vi "Server_Refresh Training Data.vi"(8 "error in":errorcluster, 11 "Index":i32) -> (0 "error out":errorcluster, 3 "Training Data":T1[](array[typedef]))   [LabVIEW 2018, in "Cloud Server.lvlib"]
uses:
  Cloud Server.lvlib
  Data Def/Server_Training Data.ctl
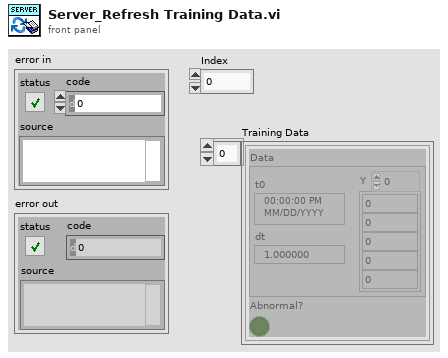
[diagram p1: front panel]
types:
  T1 = typedef "Cloud Server.lvlib/Server_Training Data.ctl" = cluster{"Data":waveform(dbl), "Abnormal?":bool}
  T2 = typedef "Cloud Server.lvlib/Server_Connection Properties.ctl" = cluster{"User Data":T3, "Data":waveform(dbl)}
  T3 = typedef "User Data.ctl" = cluster{"Name":string, "Email":string, "Phone Number":string, "User Picture":u32[][], "Last Login Time":timestamp}
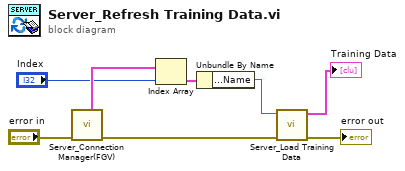
[diagram p0: block diagram]
diagram:
  n1 = call "Server_Connection Manager(FGV).vi"("error in"="error in") -> ("error out"=w5:errorcluster, "All Connection Properties"=w7:T2[])  [unwired: 6 in, 3 out]
  n2 = Index Array(array=w7, index="Index") -> (element=w4:T2)
  n3 = Unbundle By Name(w4) -> ("User Data.Name"=w3:string)
  n4 = call "Server_Load Training Data.vi"("error in"=w5, "Name"=w3) -> ("error out"=→"error out":errorcluster, "Training Data"=→"Training Data":T1[])  [unwired: 8 in]
